vi "Global_Tamb.vi"() -> ()   [LabVIEW 2019]
panel:
  out "T amb res meter":dbl
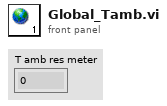
[diagram p1: front panel]
diagram:
